vi "Draw Flat Bottom Filled Triangle.vi"(4 "Fill Colour":u32(colorbox), 8 "Point 3":T1, 9 "Point 2":T1, 10 "Point 1":T1, 11 "Pixel Data in":u32[][](array[numeric])) -> (3 "Pixel Data out":u32[][](array[numeric]))   [LabVIEW 2022 SP3, in "Raster.lvlib"]
uses:
  Raster.lvlib
  Point 2D.ctl
  Method.ctl
  <vilib>/Utility/High Resolution Relative Seconds.vi
  Utility/Utility.lvlib
panel:
  out "Delta Time [s]":dbl format="%.3p"
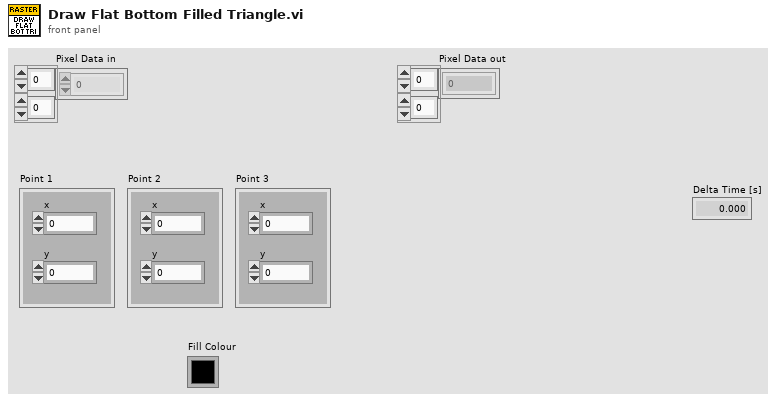
[diagram p1: front panel]
types:
  T1 = typedef "Raster.lvlib/Point 2D.ctl" = cluster{"x":i32, "y":i32}
  T2 = typedef "Raster.lvlib/Method.ctl" = enum16{"Per item", "Row", "Replace Array Subset", "MoveBlock", " MoveBlock2 "}
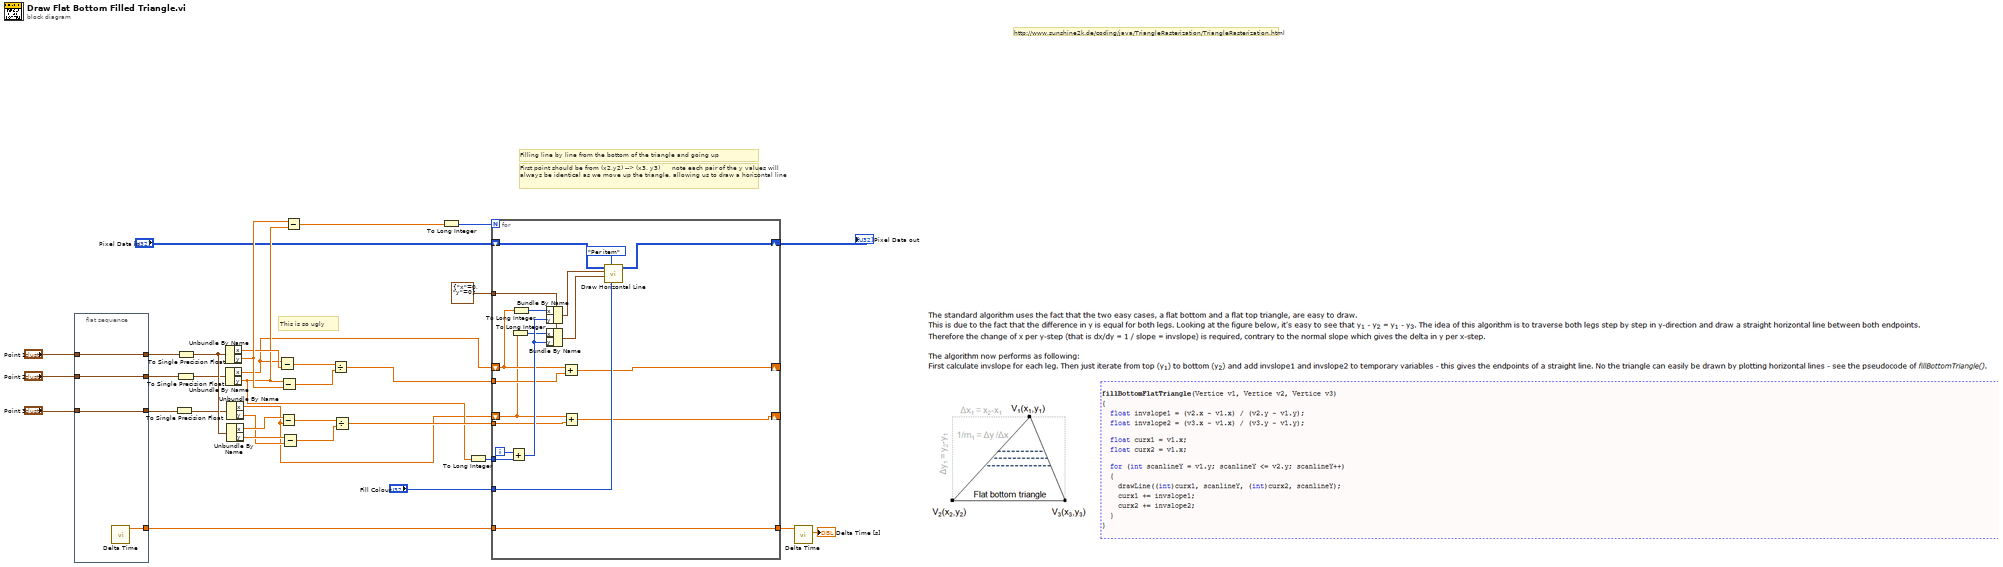
[diagram p0: block diagram]
diagram:
  # "This is so ugly"
  # "First point should be from (x2,y2) --> (x3, y3)      note each pair of the y values will always be identical as we move up the triangle, allowing us to draw a horizontal line"
  # "Filling line by line from the bottom of the triangle and going up"
  # "http://www.sunshine2k.de/coding/java/TriangleRasterization/TriangleRasterization.html"
  n1 = flat-sequence {
    tunnel: "Point 3" -> [w37]
    tunnel: [w37] -> w10
    tunnel: [w36] -> w9
    tunnel: "Point 2" -> [w36]
    tunnel: [w35] -> w7
    tunnel: "Point 1" -> [w35]
    tunnel: [w34] -> w5
    frame #0 {
      n2 = call "Delta Time.vi"() -> ("Relative Seconds Out"=w34:dbl)  [unwired: 10 in, 1 out]
    }
  }
  n3 = To Single Precision Float(number=w10) -> (single precision float=w27:cluster{"x":sgl, "y":sgl})
  n4 = To Single Precision Float(number=w9) -> (single precision float=w28:cluster{"x":sgl, "y":sgl})
  n5 = To Single Precision Float(number=w7) -> (single precision float=w29:cluster{"x":sgl, "y":sgl})
  n6 = Unbundle By Name(w29) -> ("x"=w18:sgl, "y"=w22:sgl)
  n7 = Unbundle By Name(w28) -> ("x"=w16:sgl, "y"=w17:sgl)
  n8 = Unbundle By Name(w27) -> ("x"=w14:sgl, "y"=w15:sgl)
  n9 = Unbundle By Name(w29) -> ("x"=w30:sgl, "y"=w32:sgl)
  n10 = Subtract(x=w16, y=w18) -> (x-y=w33:sgl)
  n11 = Subtract(x=w30, y=w14) -> (x-y=w31:sgl)
  n12 = Subtract(x=w17, y=w22) -> (x-y=w25:sgl)
  n13 = Subtract(x=w32, y=w15) -> (x-y=w26:sgl)
  n14 = Subtract(x=w22, y=w17) -> (x-y=w13:sgl)
  n15 = Divide(x=w33, y=w25) -> (x/y=w20:sgl)
  n16 = Divide(x=w31, y=w26) -> (x/y=w19:sgl)
  n17 = To Long Integer(number=w13) -> (32bit integer=w12:i32)
  n18 = To Long Integer(number=w17) -> (32bit integer=w21:i32)
  n19 = for {
    N: w12 -> [_]
    tunnel: T1 {"x"=0, "y"=0} ("Point 1") -> [w56]
    tunnel: "Fill Colour" -> [w53]
    shift-right: [w44] -> _
    shift-left: w16 -> [w47]
    shift-right: [w45] -> _
    shift-left: w14 -> [w42]
    tunnel: w21 -> [w49]
    tunnel: w20 -> [w46]
    tunnel: w19 -> [w43]
    tunnel: [w41] -> w4
    tunnel: w5 -> [w41]
    shift-right: [w39] -> w1
    shift-left: "Pixel Data in" -> [w40]
    i -> [w51]
    n20 = Add(x=w51, y=w49) -> (x+y=w50:i32)
    n21 = To Long Integer(number=w42) -> (32bit integer=w48:i32)
    n22 = To Long Integer(number=w47) -> (32bit integer=w52:i32)
    n23 = Bundle By Name(cluster=w56, "x"=w52, "y"=w50) -> (w55:T1)
    n24 = Bundle By Name(cluster=w56, "x"=w48, "y"=w50) -> (w54:T1)
    n25 = Add(x=w47, y=w46) -> (x+y=w44:sgl)
    n26 = Add(x=w42, y=w43) -> (x+y=w45:sgl)
    n27 = call "Draw Horizontal Line.vi"("Colour"=w53, "Method"=Method."Per item", "Point 2"=w54, "Point 1"=w55, "Pixel Data in"=w40) -> ("Pixel Data out"=w39:u32[][])  [unwired: 6 in]
  }
  "Pixel Data out" <- w1
  n28 = call "Delta Time.vi"("Relative Seconds In"=w4) -> ("Delta Time [s]"=→"Delta Time [s]":dbl)  [unwired: 9 in, 1 out]
